vi "Temp Function.vi"(4 "TRM":dbl=0.928 format="%.3f", 5 "TCR2":dbl=3e-07 format="%.2e", 6 "TRH":dbl=0.766 format="%.3f", 7 "TCR1":dbl=0.00205 format="%.2e", 8 "Ramb":dbl=10.08 format="%.3f", 9 "Tamb":dbl=25.0 format="%.3f", 10 "I":dbl[](array[numeric])=[0.1], 11 "V":dbl[](array[numeric])=[2.008]) -> (3 "Tamb":dbl[](array[numeric]))   [LabVIEW 2019]
doc: "This example demonstrates how to acquire a continuous amount of data (Waveform) using the DAQ device's internal clock. It also shows how to synchronize two devices for different device families (E Series, S Series, M Series, X Series, DSA, and SC Express), to simultaneously acquire the data.\n\nFor instructions on how to connect your signals to the DAQ device, refer to your device documentation."
panel:
  out "c":dbl[](array[numeric])
  out "Vcalc":dbl[](array[numeric])
  out "Rh0":dbl=0.0077212800000000005
  in  "TRH 2":dbl=25.0 format="%.3f"
  # "Heater Temperature Function"
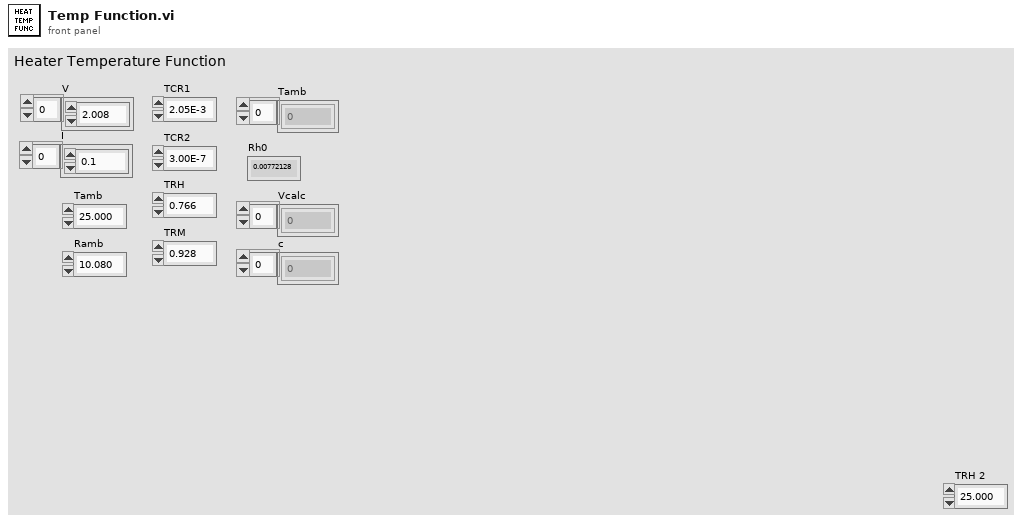
[diagram p1: front panel]
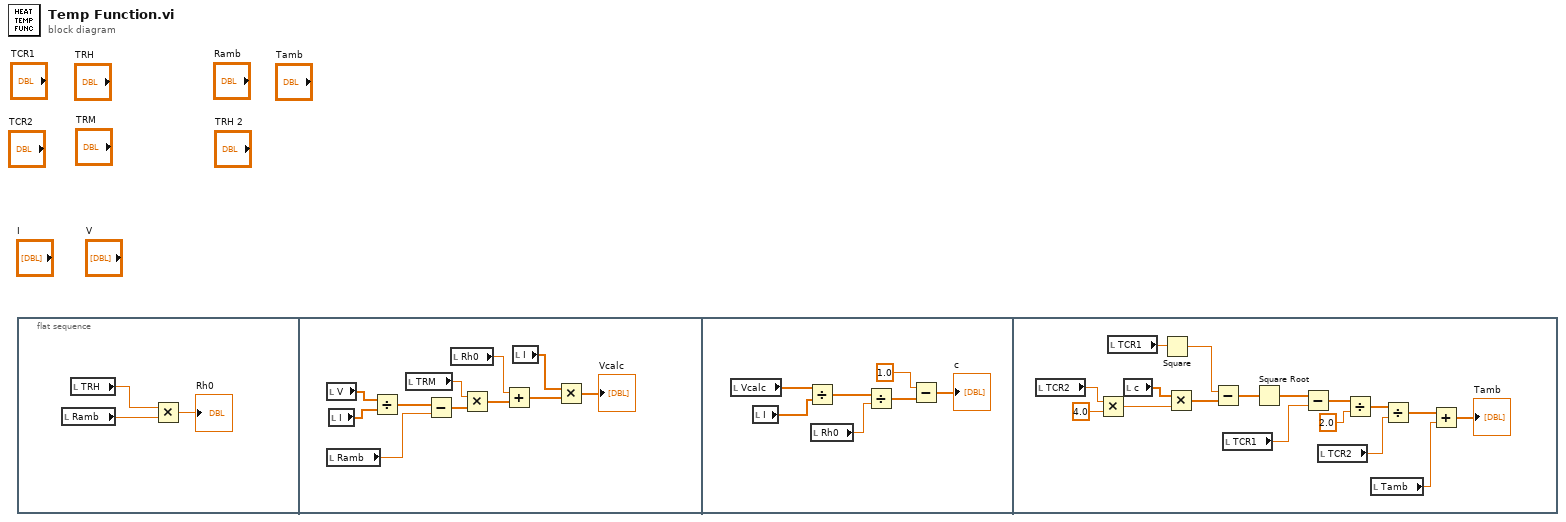
[diagram p0: block diagram]
diagram:
  n1 = flat-sequence {
    frame #0 {
      n2 = local read "Ramb"() -> (w3:dbl)
      n3 = local read "TRH"() -> (w2:dbl)
      n4 = Multiply(x=w2, y=w3) -> (x*y=→"Rh0":dbl)
    }
    frame #1 {
      n5 = local read "V"() -> (w5:dbl[])
      n6 = local read "Ramb"() -> (w9:dbl)
      n7 = local read "I"() -> (w6:dbl[])
      n8 = Divide(x=w5, y=w6) -> (x/y=w7:dbl[])
      n9 = local read "TRM"() -> (w10:dbl)
      n10 = Subtract(x=w7, y=w9) -> (x-y=w8:dbl[])
      n11 = local read "Rh0"() -> (w12:dbl)
      n12 = Multiply(x=w10, y=w8) -> (x*y=w11:dbl[])
      n13 = Add(x=w12, y=w11) -> (x+y=w13:dbl[])
      n14 = local read "I"() -> (w14:dbl[])
      n15 = Multiply(x=w14, y=w13) -> (x*y=→"Vcalc":dbl[])
    }
    frame #2 {
      n16 = local read "Vcalc"() -> (w17:dbl[])
      n17 = local read "I"() -> (w18:dbl[])
      n18 = Divide(x=w17, y=w18) -> (x/y=w19:dbl[])
      n19 = local read "Rh0"() -> (w20:dbl)
      n20 = Divide(x=w19, y=w20) -> (x/y=w21:dbl[])
      n21 = Subtract(x=1.0, y=w21) -> (x-y=→"c":dbl[])
    }
    frame #3 {
      n22 = local read "TCR2"() -> (w26:dbl)
      n23 = Multiply(x=w26, y=4.0) -> (x*y=w27:dbl)
      n24 = local read "TCR1"() -> (w25:dbl)
      n25 = local read "c"() -> (w28:dbl[])
      n26 = Square(x=w25) -> (x^2=w30:dbl)
      n27 = Multiply(x=w28, y=w27) -> (x*y=w29:dbl[])
      n28 = Subtract(x=w30, y=w29) -> (x-y=w31:dbl[])
      n29 = local read "TCR1"() -> (w33:dbl)
      n30 = Square Root(x=w31) -> (sqrt(x)=w32:dbl[])
      n31 = Subtract(x=w32, y=w33) -> (x-y=w34:dbl[])
      n32 = local read "TCR2"() -> (w36:dbl)
      n33 = Divide(x=w34, y=2.0) -> (x/y=w35:dbl[])
      n34 = local read "Tamb"() -> (w38:dbl)
      n35 = Divide(x=w35, y=w36) -> (x/y=w37:dbl[])
      n36 = Add(x=w37, y=w38) -> (x+y=→"Tamb":dbl[])
    }
  }
